vi "TCP Write Entire Buffer.vi"(8 "error in (no error)":errorcluster, 10 "data in":string, 11 "connection ID":refnum<k5>) -> (0 "error out":errorcluster, 2 "bytes written":i32, 3 "connection ID out":refnum<k5>)   [LabVIEW 2017, in "NI_FTP.lvlib"]
doc: "Writes entire buffer to a TCP connection (retrying if a Time Out Error is returned)."
uses:
  <vilib>/FTP/NI_FTP.lvlib
panel:
  in  "Num Retries":i32=10
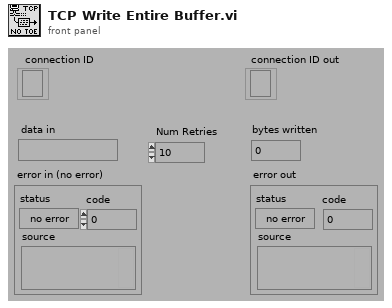
[diagram p1: front panel]
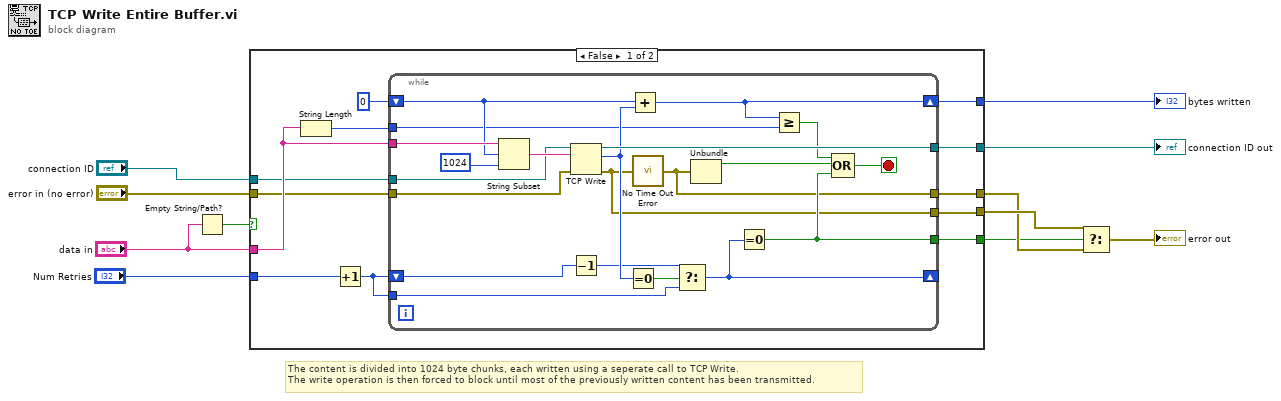
[diagram p0: block diagram]
diagram:
  # "The content is divided into 1024 byte chunks, each written using a seperate call to TCP Write.\nThe write operation is then forced to block until most of the previously written content has been transmitted."
  n1 = Empty String/Path?(string/path="data in") -> (empty?=w9:bool)
  n2 = case shown="False" w9 {
    tunnel: "data in" -> [w23 _]
    tunnel: [w19 w46] -> w5
    tunnel: [w16 w45] -> w4
    tunnel: "error in (no error)" -> [w20 w45]
    tunnel: "connection ID" -> [w21 w46]
    tunnel: [w14 _] -> w1
    tunnel: [w17 w45] -> w7
    tunnel: "Num Retries" -> [w13 _]
    tunnel: [w15 _] -> w6
    frame False {
      n3 = String Length(string=w23) -> (length=w18:i32)
      n4 = Increment(x=w13) -> (x+1=w12:i32)
      n5 = while {
        tunnel: w23 -> [w44]
        shift-right: [w30] -> w15
        shift-left: 0 -> [w32]
        tunnel: w18 -> [w29]
        tunnel: w21 -> [w42]
        tunnel: w20 -> [w41]
        tunnel: [w40] -> w19
        shift-right: [w26] -> _
        shift-left: w12 -> [w25]
        tunnel: [w35] -> w14
        tunnel: [w34] -> w17
        tunnel: [w33] -> w16
        tunnel: w12 -> [w24]
        stop <- w38 stop-if-true
        n6 = String Subset(string=w44, offset (0)=w32, length (rest)=1024) -> (substring=w43:string)
        n7 = TCP Write(connection ID=w42, data in=w43, error in (no error)=w41) -> (connection ID out=w40:refnum<k5>, bytes written=w36:i32, error out=w34:errorcluster)  [unwired: 1 out]
        n8 = Decrement(x=w25) -> (x-1=w27:i32)
        n9 = Equal To 0?(x=w36) -> (x = 0?=w37:bool)
        n10 = Add(x=w32, y=w36) -> (x+y=w30:i32)
        n11 = call <vilib>:"No Time Out Error.vi"("error in (no error)"=w34) -> ("error out"=w33:errorcluster)  [unwired: 14 out]
        n12 = Select(t=w27, s=w37, f=w24) -> (s? t:f=w26:i32)
        n13 = Unbundle(w33) -> ("status"=w39:bool)  [unwired: 2 out]
        n14 = Equal To 0?(x=w26) -> (x = 0?=w35:bool)
        n15 = Greater Or Equal?(x=w30, y=w29) -> (x >= y?=w28:bool)
        n16 = Compound Arithmetic op=OR(w28, w39, w35) -> (w38:bool)
      }
    }
    frame True {
    }
  }
  "connection ID out" <- w5
  "bytes written" <- w6
  n17 = Select(t=w7, s=w1, f=w4) -> (s? t:f=→"error out":errorcluster)
